vi "GetLogFilePath.vi"(3 "Server name":string) -> (0 "LogFolder":path, 1 "LogPath":path)   [LabVIEW 2012]
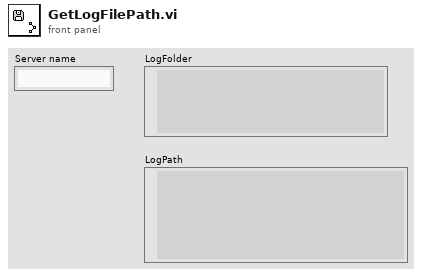
[diagram p1: front panel]
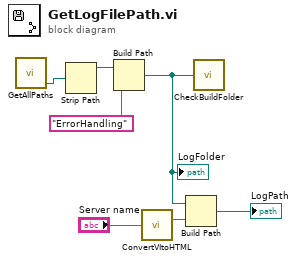
[diagram p0: block diagram]
diagram:
  n1 = call <userlib>:"GetAllPaths.vi"() -> ("Server Folder"=w4:path)  [unwired: 1 in, 2 out]
  n2 = Strip Path(path=w4) -> (stripped path=w3:path)  [unwired: 1 out]
  n3 = Build Path(base path=w3, name or relative path="ErrorHandling") -> (appended path=w5:path)
  "LogFolder" <- w5
  n4 = call <userlib>:"ConvertVItoHTML.vi"("vi name"="Server name") -> ("Htm log name"=w1:string)  [unwired: 1 out]
  n5 = Build Path(base path=w5, name or relative path=w1) -> (appended path=→"LogPath":path)
  n6 = call <userlib>:"CheckBuildFolder.vi"("appended path"=w5) -> ()  [unwired: 1 in]
